vi "is error.vi"(10 "exception":T1 {"code" format="%.0x"}) -> (2 "error!":bool)   [LabVIEW 2013, in "exception.lvlib"]
uses:
  exception.lvlib
  exception.ctl
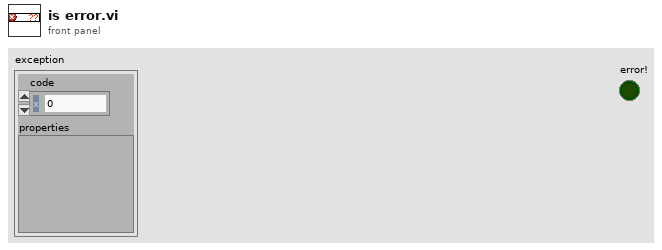
[diagram p1: front panel]
types:
  T1 = typedef "exception.lvlib/exception.ctl" = cluster{"code":i32, "properties":variant}
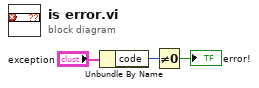
[diagram p0: block diagram]
diagram:
  n1 = Unbundle By Name("exception") -> ("code"=w2:i32)
  n2 = Not Equal To 0?(x=w2) -> (x != 0?=→"error!":bool)
